vi "openShutter.vi"(8 "error in (no error)":errorcluster, 11 "IDome in":refnum<class "IDome.lvclass">) -> (0 "error out":errorcluster, 3 "IDome out":refnum<class "IDome.lvclass">)   [LabVIEW 2016, in "IDome.lvclass"]
uses:
  IDome.lvclass
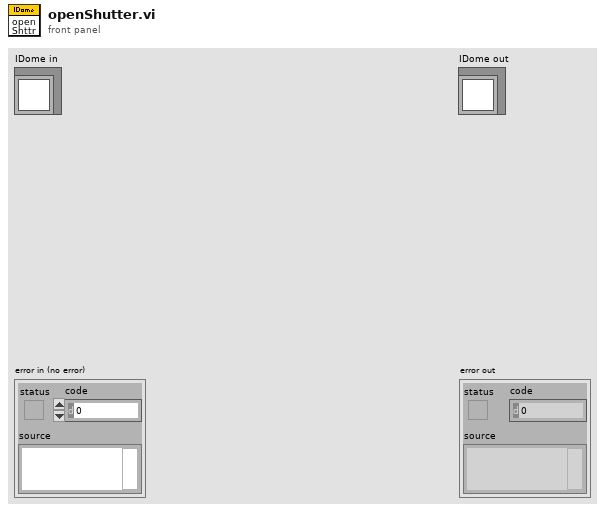
[diagram p1: front panel]
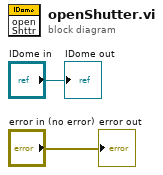
[diagram p0: block diagram]
diagram:
  "error out" <- "error in (no error)"
  "IDome out" <- "IDome in"
